vi "DispLastRow(MList).vi"(6 "显示尾行":bool, 8 "error in (no error)":errorcluster caption="错误输入（无错误）", 11 "MCListbox引用句柄":refnum<vi>) -> (0 "error out":errorcluster caption="错误输出", 3 "Ctl句柄输出":refnum<vi>)   [LabVIEW 2011]
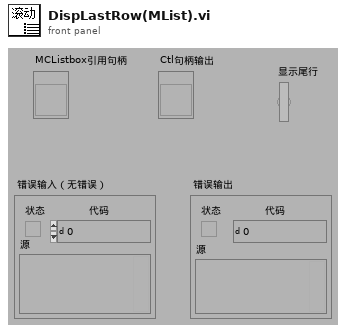
[diagram p1: front panel]
types:
  T1 = typedef "LVRowAndColumnUnsignedTypeDef.ctl" = cluster{"Row":u32, "Column":u32}
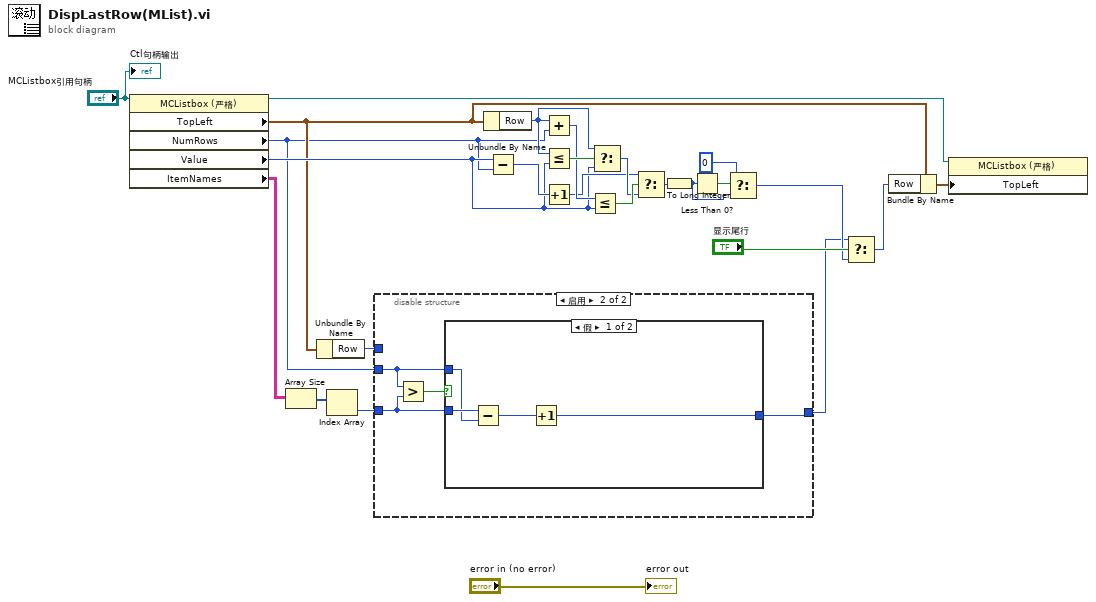
[diagram p0: block diagram]
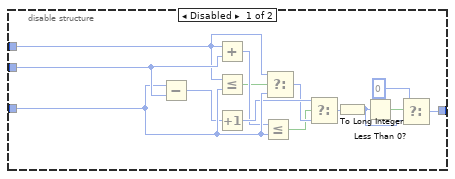
[diagram p2: hidden frame]
diagram:
  n1 = property class="MCListbox (严格)"(reference="MCListbox引用句柄") -> (reference out=w18:refnum<vi>, "TopLeft"=w8:T1, "NumRows"=w7:u32, "Value"=w11:i32, "ItemNames"=w10:string[][])  [unwired: 1 in, 1 out]
  n2 = Array Size(array=w10) -> (size(s)=w9:i32[])
  n3 = Unbundle By Name(w8) -> ("Row"=w1:u32)
  n4 = Index Array(array=w9) -> (element=w2:i32)  [unwired: 1 in]
  n5 = disable-structure shown="启用" {
    disable-tunnel: w7 -> [w40 w43]
    disable-tunnel: [w39 w41] -> w4
    disable-tunnel: w2 -> [w38 w42]
    disable-tunnel: w1 -> [w28 _]
    frame Disabled {
      n6 = Subtract(x=w38, y=w40) -> (x-y=w32:u32)
      n7 = Add(x=w28, y=w40) -> (x+y=w29:u32)
      n8 = Less Or Equal?(x=w28, y=w38) -> (x <= y?=w27:bool)
      n9 = Increment(x=w32) -> (x+1=w33:u32)
      n10 = Less Or Equal?(x=w29, y=w38) -> (x <= y?=w30:bool)
      n11 = Select(t=w28, s=w27, f=w38) -> (s? t:f=w31:u32)
      n12 = Select(t=w33, s=w30, f=w31) -> (s? t:f=w34:u32)
      n13 = To Long Integer(number=w34) -> (32bit integer=w36:i32)
      n14 = Less Than 0?(x=w36) -> (x < 0?=w35:bool)
      n15 = Select(t=0, s=w35, f=w36) -> (s? t:f=w39:i32)
    }
    frame Enabled {
      n16 = Greater?(x=w43, y=w42) -> (0:w44:bool)
      n17 = case shown="假" w44 {
        tunnel: w43 -> [w47 _]
        tunnel: w42 -> [w48 _]
        tunnel: [w45 _] -> w41
        frame False {
          n18 = Subtract(x=w48, y=w47) -> (x-y=w46:u32)
          n19 = Increment(x=w46) -> (x+1=w45:u32)
        }
        frame True {
        }
      }
    }
  }
  n20 = Unbundle By Name(w8) -> ("Row"=w25:u32)
  n21 = Subtract(x=w11, y=w7) -> (x-y=w21:u32)
  n22 = Add(x=w25, y=w7) -> (x+y=w24:u32)
  n23 = Less Or Equal?(x=w25, y=w11) -> (x <= y?=w26:bool)
  n24 = Increment(x=w21) -> (x+1=w20:u32)
  n25 = Less Or Equal?(x=w24, y=w11) -> (x <= y?=w23:bool)
  n26 = Select(t=w25, s=w26, f=w11) -> (s? t:f=w22:u32)
  n27 = Select(t=w20, s=w23, f=w22) -> (s? t:f=w15:u32)
  n28 = To Long Integer(number=w15) -> (32bit integer=w13:i32)
  n29 = Less Than 0?(x=w13) -> (x < 0?=w14:bool)
  n30 = Select(t=0, s=w14, f=w13) -> (s? t:f=w5:i32)
  n31 = Select(t=w4, s="显示尾行", f=w5) -> (s? t:f=w3:u32)
  n32 = Bundle By Name(cluster=w8, "Row"=w3) -> (w19:T1)
  n33 = property class="MCListbox (严格)"(reference=w18, "TopLeft"=w19) -> ()  [unwired: 1 in, 2 out]
  "Ctl句柄输出" <- "MCListbox引用句柄"
  "error out" <- "error in (no error)"
